vi "Check Default Response.vi"(8 "Failed Response in":refnum<class "Response.lvclass">, 11 "Success Response in":refnum<class "Response.lvclass">) -> (0 "Failed Response":refnum<class "Response.lvclass">, 3 "Success Response":refnum<class "Response.lvclass">)   [LabVIEW 2020, in "OAuth2.lvlib" / "OAuth2.lvclass"]
uses:
  OAuth2.lvclass
  OAuth2.lvclass/OAuth2.ctl
  <vilib>/IlluminatedG/IG HTTP Utils/HTTP Utils/Response/Response.lvclass
  OAuth2.lvlib
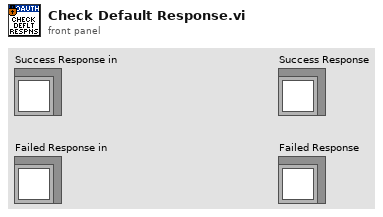
[diagram p1: front panel]
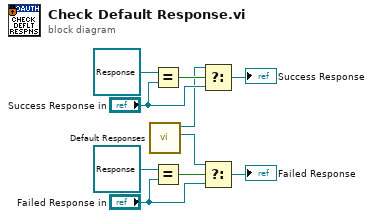
[diagram p0: block diagram]
diagram:
  n1 = call "Default Responses.vi"() -> ("Default Failed Response"=w3:refnum<class "Response.lvclass">, "Default Success Response"=w4:refnum<class "Response.lvclass">)  [unwired: 10 in]
  n2 = Equal?(x=refnum<class "Response.lvclass"> refnum, y="Success Response in") -> (x = y?=w7:bool)
  n3 = Equal?(x=refnum<class "Response.lvclass"> refnum, y="Failed Response in") -> (x = y?=w8:bool)
  n4 = Select(t=w4, s=w7, f="Success Response in") -> (s? t:f=→"Success Response":refnum<class "Response.lvclass">)
  n5 = Select(t=w3, s=w8, f="Failed Response in") -> (s? t:f=→"Failed Response":refnum<class "Response.lvclass">)
